vi "MasterAquisitionFile_IOS_Optogenetics_Test2.vi"() -> ()   [LabVIEW 2018]
uses:
  <vilib>/vision/driver/IMAQdx.llb/IMAQdx Camera Control Mode.ctl
  <vilib>/vision/driver/IMAQdx.llb/IMAQdx Acquisition Mode.ctl
  <vilib>/userdefined/High Color/IMAQdx.ctl
  <vilib>/vision/driver/IMAQdx.llb/IMAQdx Buffer Number Mode.ctl
  <vilib>/DAQmx/write.llb/DAQmx Write (Digital 1D Wfm NChan NSamp).vi
  <vilib>/DAQmx/read.llb/DAQmx Read (Analog 1D Wfm NChan NSamp).vi
  <vilib>/Waveform/DWDTOps.llb/DWDT Digital to Boolean Array.vi
  <vilib>/DAQmx/create/channels.llb/DAQmx Create Channel (CO-Pulse Generation-Frequency).vi
  <vilib>/DAQmx/configure/timing.llb/DAQmx Timing (Implicit).vi
  <vilib>/DAQmx/create/channels.llb/DAQmx Create Channel (AI-Voltage-Basic).vi
  <vilib>/DAQmx/configure/timing.llb/DAQmx Timing (Sample Clock).vi
  <vilib>/DAQmx/configure/trigger.llb/DAQmx Start Trigger (Digital Edge).vi
  <vilib>/DAQmx/create/channels.llb/DAQmx Create Channel (DO-Digital Output).vi
  <vilib>/Waveform/DWDTOps.llb/DWDT Uncompress Digital.vi
  <vilib>/DAQmx/miscellaneous.llb/DAQmx Fill In Error Info.vi
  <vilib>/vision/driver/NI_Vision_Acquisition_Software.lvlib
  <resource>/objmgr/imaqdx.rc
  <resource>/objmgr/daqmx.rc
panel:
  out "Samples Written to Channel":dbl
  out "LED":bool
  out "Auditory":bool
  out "RPad":bool
  out "LPad":bool
  out "Finished":bool
  in  "Generate Stimuli":bool=TRUE
  in  "Sol Stim Parameters":cluster{"Fs":dbl, "Samples":dbl}
  in  "LED Stim Parameters":cluster{"Fs":dbl, "Samples":dbl}
  in  "Sol Duty Cycle (%)":dbl=10.0
  in  "Sol Freq":dbl=1.0
  in  "Sol Dur (s)":dbl=1.0
  in  "LED Duty Cycle (%)":dbl=10.0
  in  "LED Freq":dbl=10.0
  in  "LED Dur (s)":dbl=2.0
  out "Stimulus Order":digitalwaveform[](graph)=[{"t0"=timestamp(0 s since 1904-01-01), "dt"=5e-05, "Y"={"transitions"=[], "data"=array18000000x1[18000000 elements]}}, {"t0"=timestamp(0 s since 1904-01-01), "dt"=5e-05, "Y"={"transitions"=[], "data"=array18000000x1[18000000 elements]}}, {"t0"=timestamp(0 s since 1904-01-01), "dt"=5e-05, "Y"={"transitions"=[], "data"=array18000000x1[18000000 elements]}}, {"t0"=timestamp(0 s since 1904-01-01), "dt"=5e-05, "Y"={"transitions"=[], "data"=array18000000x1[18000000 elements]}}]
  out "Solenoid Stim":digitalwaveform(graph)={"t0"=timestamp(0 s since 1904-01-01), "dt"=5e-05, "Y"={"transitions"=[], "data"=array20000x1[20000 elements]}}
  in  "Trial Offset (s)":dbl=15.0
  in  "Interstim (s)":dbl=30.0
  in  "Right Pad":dbl=1.0
  in  "Left Pad":dbl=1.0
  in  "Auditory":dbl=1.0
  in  "LED":dbl
  out "Dev2 Samples":i32=526603
  out "Dev2 Analog":bool=TRUE
  in  "Dev2 Analog Channels":string[](array[string])=["LD_BackScatter", "LD_Flow", "Opto_LED", "RPadSol", "AudSol", "Hippocampus", "EMG", "Cortical_RH"]
  out "?":T1(plugin-control)
  out "?":T1(plugin-control)
  out "?":T1(plugin-control)
  out "?":T1(plugin-control)
  in  "stop":bool
  out "CBV Cam":bool=TRUE
  out "Pupil Cam":bool=TRUE
  out "Whisk Cam":bool=TRUE
  out "Web Cam":bool=TRUE
  out "Dev1 Analog":bool=TRUE
  out "Web Cam Fs":dbl(knob)=29.14753443801158 scale=0.0..200.0
  out "CBV Cam":dbl(knob)=30.019685039370078 scale=0.0..200.0
  out "Whisk Cam Fs":dbl(knob)=150.04985044865404 scale=0.0..200.0
  out "Last Whisk\nBuffer 2":u32=789
  out "Pupil Cam Fs":dbl(knob)=29.985007496251875 scale=0.0..200.0
  out "Dropped 2":u32(slide) caption="Pupil Cam" scale=0.0..99.0
  in  "Exposure Time (microsec)":string="10000"
  out "Dev1 Samples":i32=526592
  in  "Dev1 Analog Channels":string[](array[string])=["Cortical_LH", "Force_Sensor", "LPadSol", "RPadSol", "AudSol", "Hippocampus", "EMG", "Cortical_RH"]
  in  "Analog Acquisition":cluster{"Analog Fs":u16}={"Analog Fs"=20000} {"Analog Fs" format="%0.0f"}
  in  "Sampling Rates":T2={"CBV Cam Fs"=30, "Whisk Cam Fs"=150, "Web Cam Fs"=15, "Pupil Cam Fs"=30}
  out "Notes Size":i32=8
  out "Notes Reversed":string[](array[string])=["Experimenter", "Animal ID", "Hemisphere", "Solenoid PSI", "Isoflurane time", "Session ID", "Amplifier Gain", "LED power (mW)"]
  out "Notes Array":string[](array[string])=["LED power (mW)", "Amplifier Gain", "Session ID", "Isoflurane time", "Solenoid PSI", "Hemisphere", "Animal ID", "Experimenter"]
  in  "Notes:":T3={"Experimenter"="Kevin", "Animal ID"="T182", "Hemisphere"="Both", "Solenoid PSI"="10", "Isoflurane time"="1030", "Session ID"="Imaging Session Two", "Amplifier Gain"="10000", "LED power (mW)"="0"}
  in  "Target Path":path=path "D:/T182/Imaging Session 2 - 20 Apr. 2021" caption="Final Save Location"
  out "Dropped":u32(slide) caption="Whisk Cam" scale=0.0..999.0
  out "Filename":string="210420_10_44_31"
  out "CBV Camera":bool
  out "Time Elapsed (Min)":cluster{dbl, dbl}(slide)={15.0, 0.43888776} scale=0.0..15.0 scale format="%#_2g"
  in  "Time (min)":dbl(knob)=15.0 min=0.5 max=20.0 step=0.5 scale=0.0..20.0 scale format="%#_2g"
  in  "Temp Path":path=path "D:/LabVIEW Streamed Data" caption="Temporary Path for Streamed Data"
  out "Last CBV\nBuffer":i32=789
  out "Last Whisk\nBuffer":u32=3948
  # "Stimuli"
  # "LPAD"
  # "RPAD"
  # "AUD"
  # "LED"
  # "Ratio"
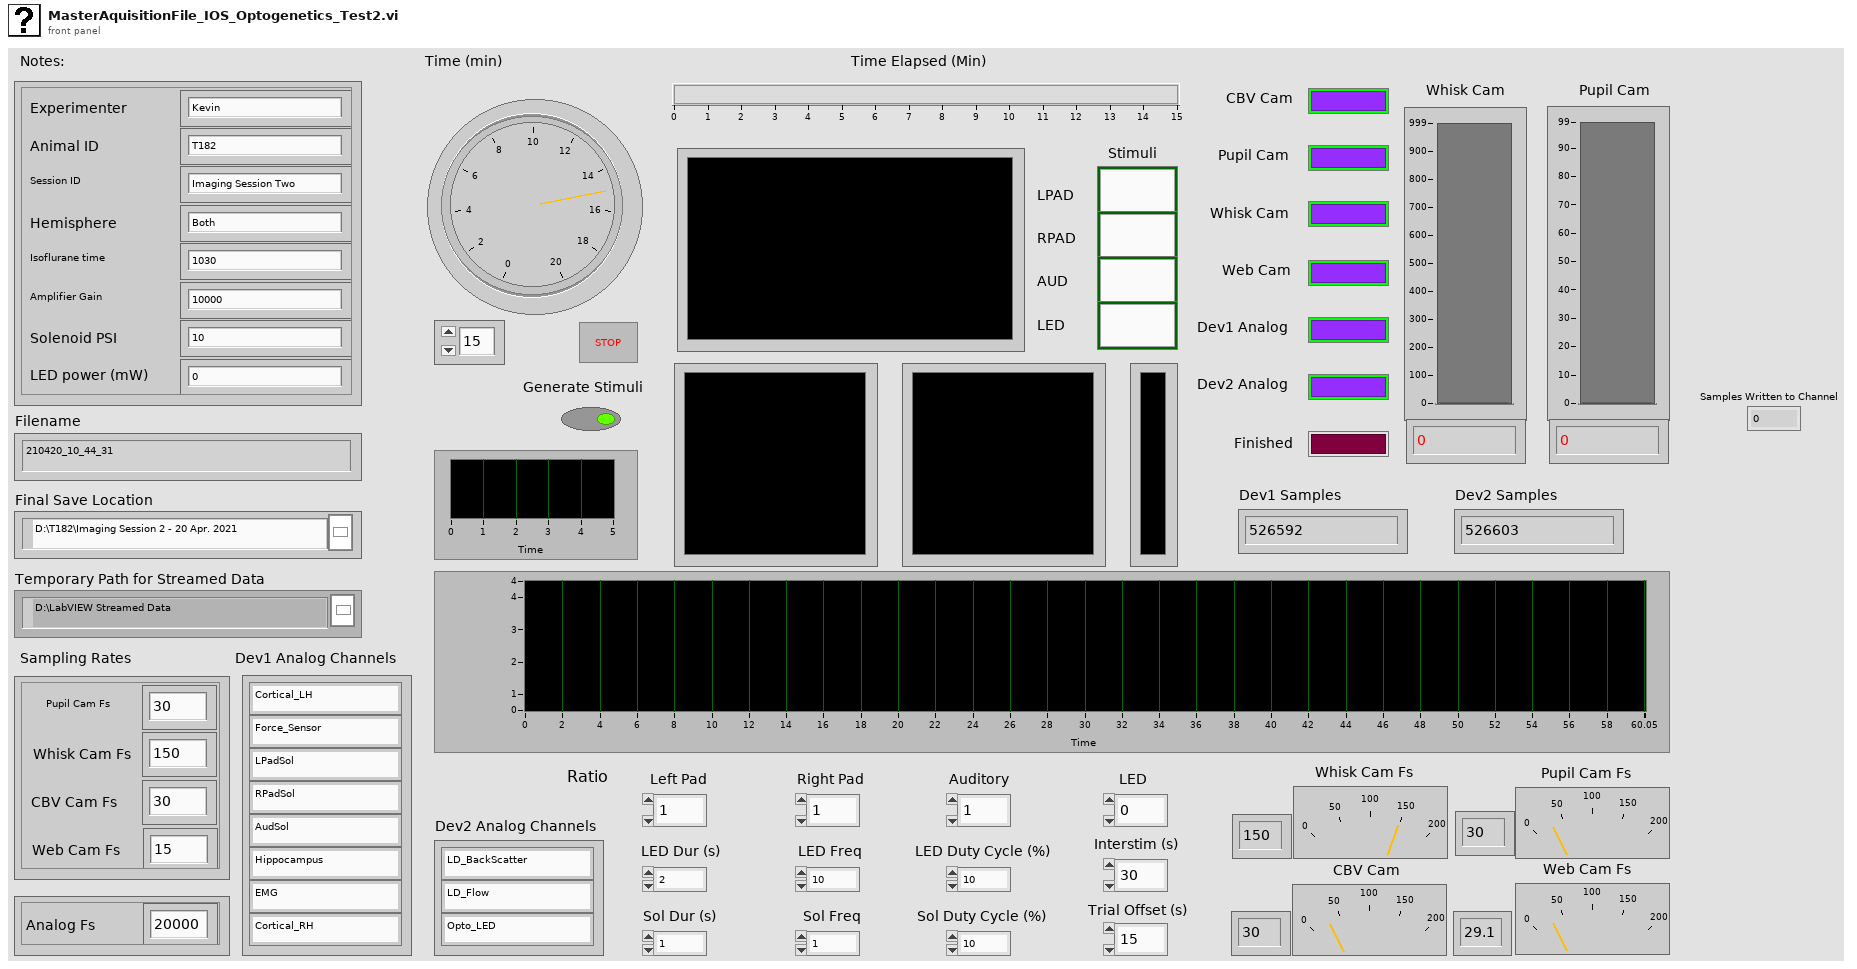
[diagram p1: front panel]
types:
  T1 = typedef "IMAQ Image.ctl" = refnum<image>
  T2 = cluster{"CBV Cam Fs":u16, "Whisk Cam Fs":u16, "Web Cam Fs":u16, "Pupil Cam Fs":u16}
  T3 = cluster{"Experimenter":string, "Animal ID":string, "Hemisphere":string, "Solenoid PSI":string, "Isoflurane time":string, "Session ID":string, "Amplifier Gain":string, "LED power (mW)":string}
  T4 = typedef "IMAQdx.ctl" = refnum<k21>
  T5 = enum16{"open", "open or create", "create or replace", "create", "open (read-only)"}
  T6 = enum16{"open", "replace", "create", "open or create", "replace or create", "replace or create with confirmation"}
  T7 = typedef "Image Type" = u32
  T8 = typedef "NI_Vision_Acquisition_Software.lvlib/IMAQdx Acquisition Mode.ctl" = enum32{"One Shot", "Continuous"}
  T9 = typedef "NI_Vision_Acquisition_Software.lvlib/IMAQdx Camera Control Mode.ctl" = enum32{"Controller", "Listener"}
  T10 = typedef "IMAQ AVI2 Refnum.ctl" = refnum<k20>
  T11 = enum16{"big-endian, network order", "native, host order", "little-endian"}
  T12 = typedef "NI_Vision_Acquisition_Software.lvlib/IMAQdx Buffer Number Mode.ctl" = enum32{"Next", "Last", "Buffer Number", "Every", "Last New"}
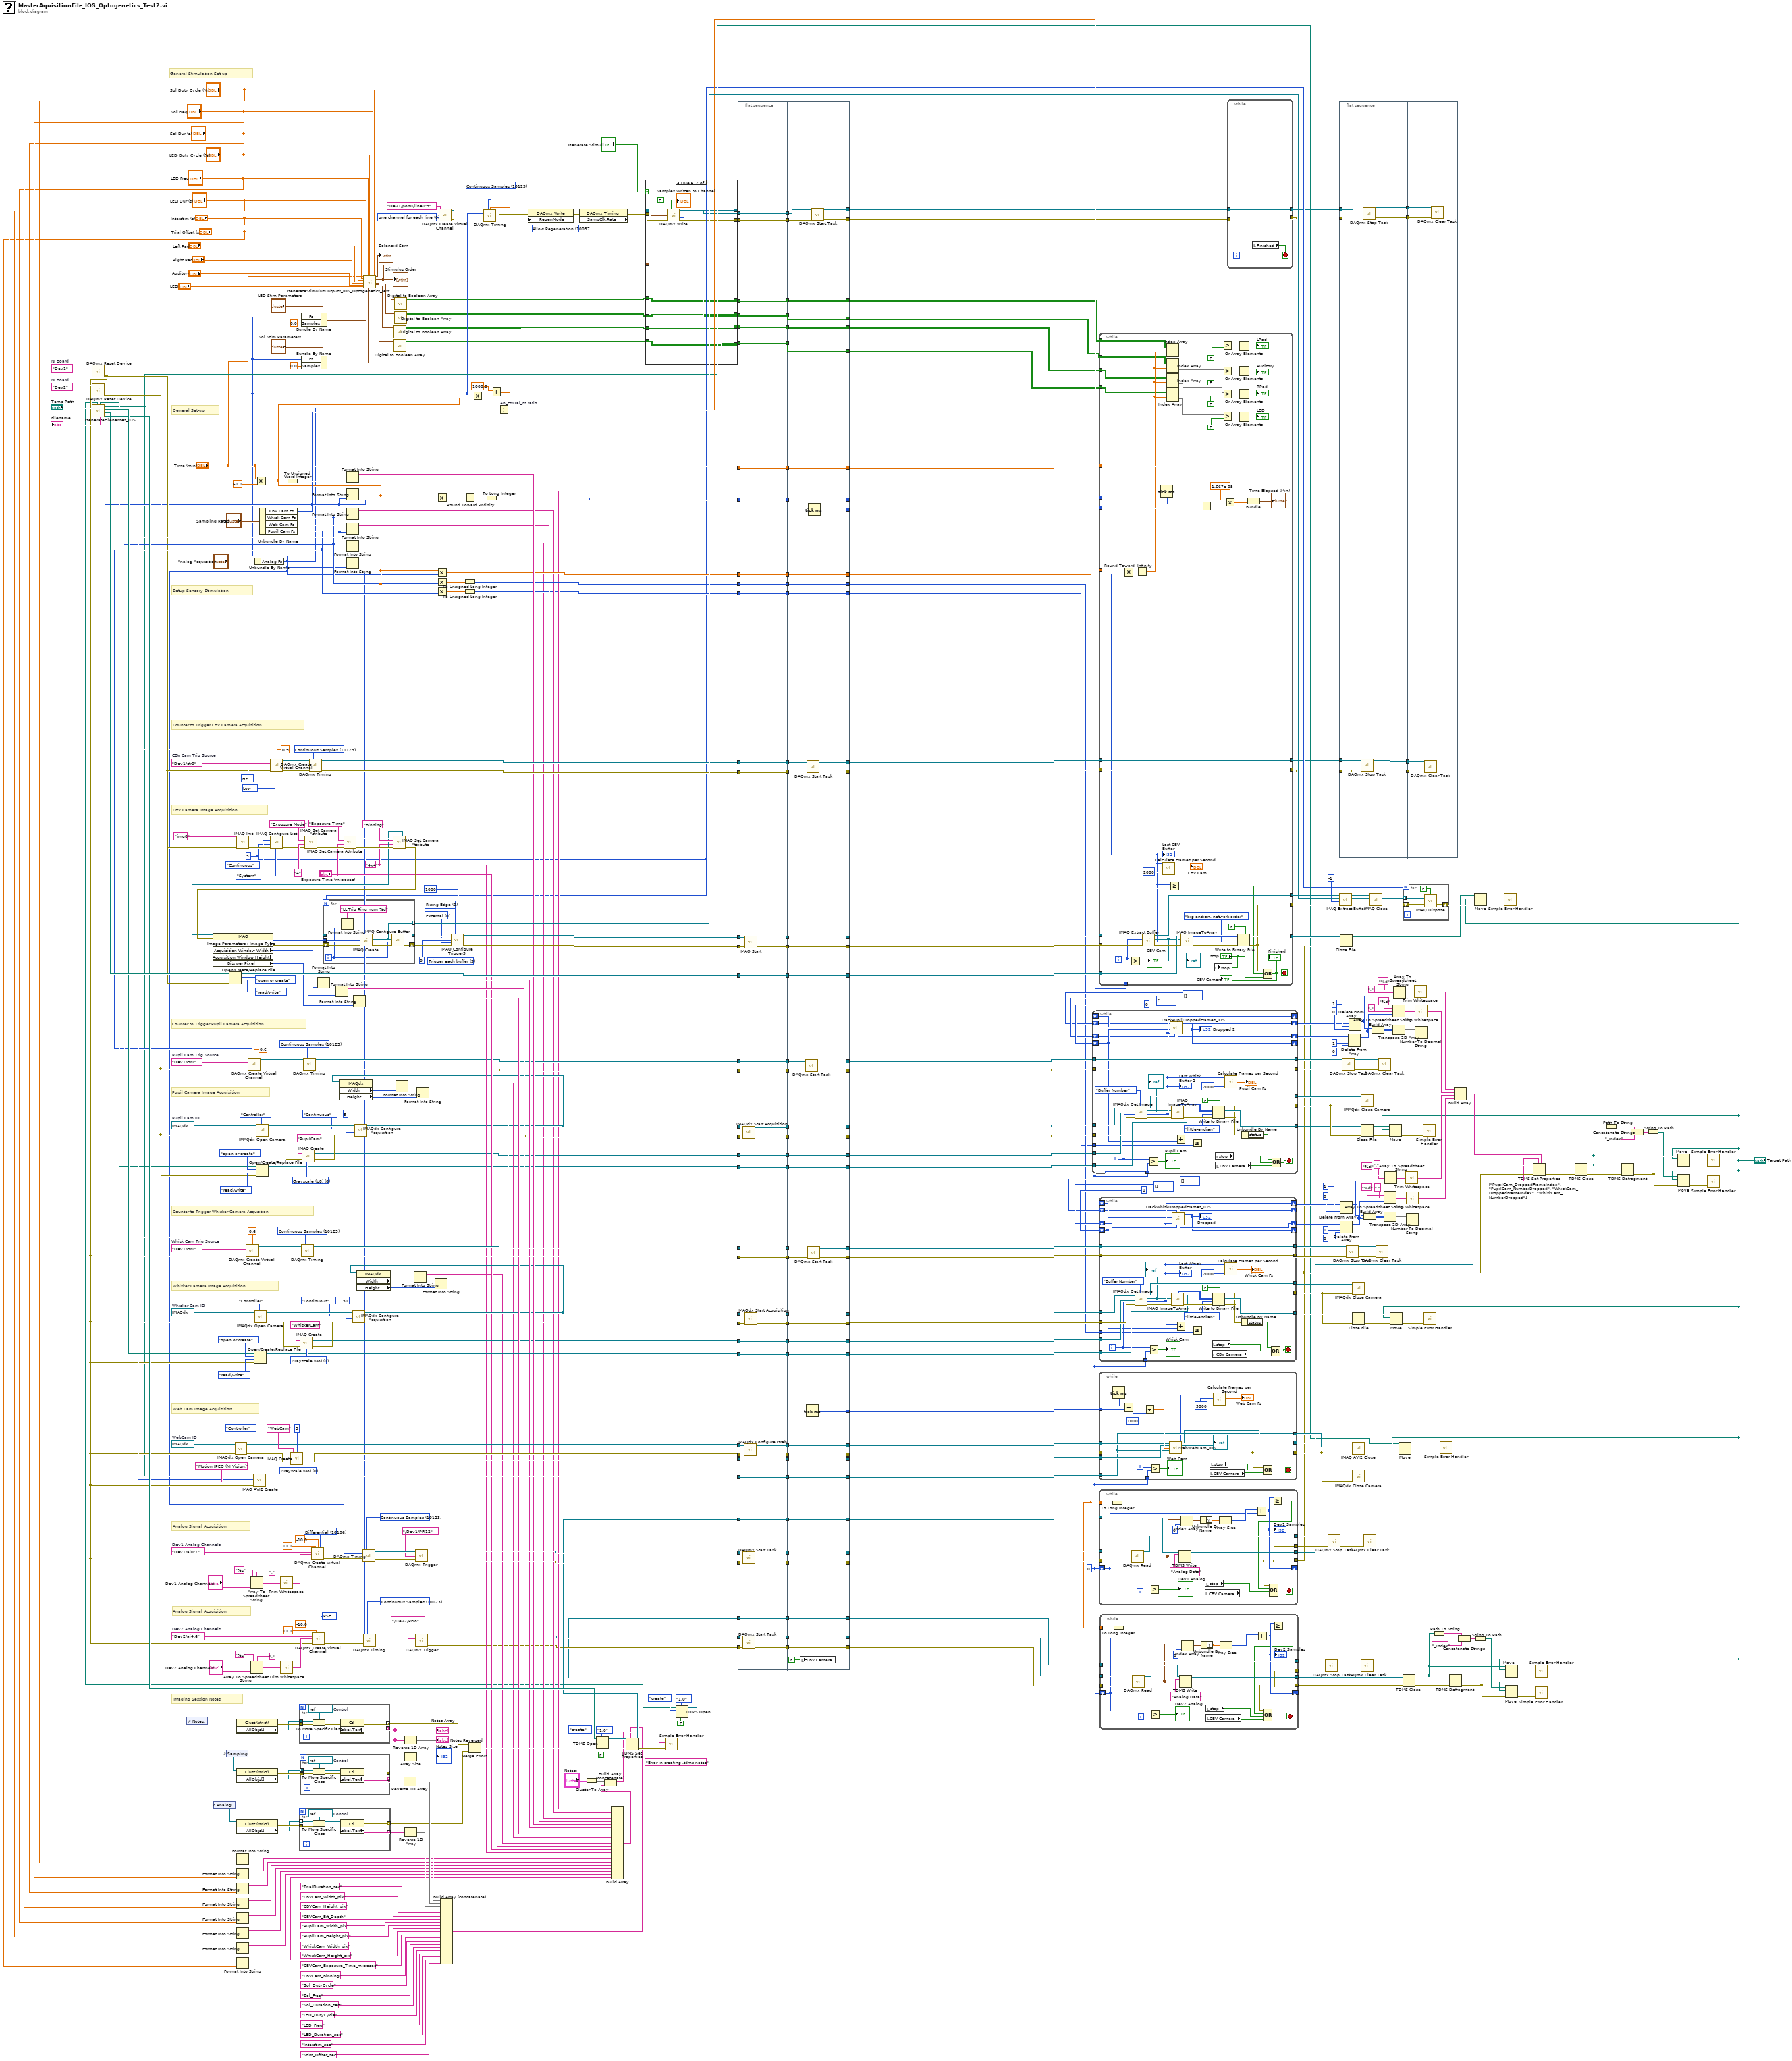
[diagram p0: block diagram]
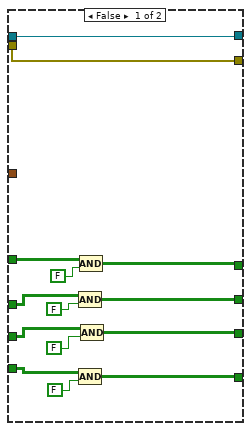
[diagram p2: hidden frame]
diagram:
  w35 = 10097 items=["Allow Regeneration"=10097, "Do Not Allow Regeneration"=10158] ("RegenMode")
  w36 = 10123 items=["Finite Samples"=10178, "Continuous Samples"=10123, "Hardware Timed Single Point"=12522] ("sample mode")
  w39 = 0 items=["one channel for each line", "one channel for all lines"] ("line grouping")
  w135 = tag "Dev2/ai4:6"  # Dev2 Analog Channels
  w315 = tag "Dev1/ai0:7"  # Dev1 Analog Channels
  w318 = T4 "cam0"  # WebCam ID
  w296 = T4 "cam1"  # Whisker Cam ID
  w488 = tag "Dev1/ctr1"  # Whisk Cam Trig Source
  w233 = T4 "cam2"  # Pupil Cam ID
  w238 = tag "Dev1/ctr0"  # Pupil Cam Trig Source
  w462 = tag "Dev1/ctr0"  # CBV Cam Trig Source
  w139 = 10123 items=["Finite Samples"=10178, "Continuous Samples"=10123, "Hardware Timed Single Point"=12522] ("sample mode")
  w142 = 10083 items=["default"=-1, "RSE"=10083, "NRSE"=10078, "Differential"=10106, "Pseudodifferential"=12529] ("input terminal configuration")
  w156 = tag "Dev2"  # NI Board
  w234 = 10123 items=["Finite Samples"=10178, "Continuous Samples"=10123, "Hardware Timed Single Point"=12522] ("sample mode")
  w241 = T7 0 items=["Grayscale (U8)", "Grayscale (I16)", "Grayscale (SGL)", "Complex (CSG)", "RGB (U32)", "HSL (U32)", "RGB (U64)", "Grayscale (U16)"] ("Image Type")
  w223 = "4x4" ("Attribute Value")
  w94 = 0
  w397 = 10123 items=["Finite Samples"=10178, "Continuous Samples"=10123, "Hardware Timed Single Point"=12522] ("sample mode")
  w400 = 10106 items=["default"=-1, "RSE"=10083, "NRSE"=10078, "Differential"=10106, "Pseudodifferential"=12529] ("input terminal configuration")
  w449 = T7 0 items=["Grayscale (U8)", "Grayscale (I16)", "Grayscale (SGL)", "Complex (CSG)", "RGB (U32)", "HSL (U32)", "RGB (U64)", "Grayscale (U16)"] ("Image Type")
  w469 = u32 0 items=["Rising Edge", "Falling Edge"] ("Trigger Polarity")
  w472 = u32 0 items=["External"=0, "RTSI"=1, "ISO In"=2, "Scaled Encoder"=5] ("Trigger Type")
  w463 = tag "Dev1"  # NI Board
  w464 = 10123 items=["Finite Samples"=10178, "Continuous Samples"=10123, "Hardware Timed Single Point"=12522] ("sample mode")
  w467 = 10373 items=["Hz"=10373] ("units")
  w468 = 10214 items=["High"=10192, "Low"=10214] ("idle state")
  w32 = u32 5 ("Number of Buffers")
  w470 = u32 3 items=["Disabled", "Trigger start of acquisition", "Trigger start of each buffer list", "Trigger each buffer", "Trigger each line (linescan)", "Trigger end of acquisition"] ("Action")
  w484 = 10123 items=["Finite Samples"=10178, "Continuous Samples"=10123, "Hardware Timed Single Point"=12522] ("sample mode")
  w491 = T7 0 items=["Grayscale (U8)", "Grayscale (I16)", "Grayscale (SGL)", "Complex (CSG)", "RGB (U32)", "HSL (U32)", "RGB (U64)", "Grayscale (U16)"] ("Image Type")
  # "General Stimulation Set-up"
  # "Analog Signal Acquisition"
  # "General Set-up"
  # "Pupil Camera Image Acquisition"
  # "Counter to Trigger Pupil Camera Acquisition"
  # "Whisker Camera Image Acquisition"
  # "Imaging Session Notes"
  # "Setup Sensory Stimulation"
  # "CBV Camera Image Acquisition"
  # "Counter to Trigger CBV Camera Acquisition"
  # "Counter to Trigger Whisker Camera Acqusition"
  # "Web Cam Image Acquisition"
  # "Analog Signal Acquisition"
  n1 = call <vilib>:"DAQmx Reset Device.vi"("device in"=w463) -> ("error out"=w128:errorcluster)  [unwired: 14 in]
  n2 = call <vilib>:"DAQmx Reset Device.vi"("device in"=w156) -> ("error out"=w155:errorcluster)  [unwired: 14 in]
  n3 = call "GenerateFilenames_IOS.vi"("path"="Temp Path") -> ("TDMS Path"=w340:path, "Dalsa Path"=w456:path, "Basler Path"=w452:path, "WebCam Path"=w79:path, "Analog file name"=→"Filename":string, "Basler2 Path"=w232:path, "TDMS Path 2"=w96:path)  [unwired: 3 in, 1 out]
  n4 = control-ref of="Notes:"() -> (w345:refnum<vi>)
  n5 = control-ref of="Analog Acquisition"() -> (w323:refnum<vi>)
  n6 = control-ref of="Sampling Rates"() -> (w324:refnum<vi>)
  n7 = Open/Create/Replace File(file path (use dialog)=w456, error in=w128, operation (0:open)=T6."open or create", access (0:read/write)=enum16{"read/write", "read-only", "write-only"}."read/write") -> (refnum out=w401:refnum<file>)  [unwired: 2 in, 2 out]
  n8 = call <vilib>:"IMAQdx Open Camera.vi"("Camera Control Mode"=IMAQdx_Camera_Control_Mode."Controller", "error in"=w128, "Session In"=w318) -> ("error out"=w445:errorcluster, "Session Out"=w443:T4)  [unwired: 7 in]
  n9 = property class="Clust (strict)"(reference=w345) -> (error out=w348:errorcluster, "AllObjs[]"=w258:refnum<vi>[])  [unwired: 1 in, 1 out]
  n10 = property class="Clust (strict)"(reference=w324) -> (error out=w343:errorcluster, "AllObjs[]"=w259:refnum<vi>[])  [unwired: 1 in, 1 out]
  n11 = property class="Clust (strict)"(reference=w323) -> (error out=w322:errorcluster, "AllObjs[]"=w257:refnum<vi>[])  [unwired: 1 in, 1 out]
  n12 = call <vilib>:"IMAQ Init.vi"("error in (no error)"=w128, "Interface Name"="img0") -> ("error out"=w482:errorcluster, "IMAQ Session Out"=w483:refnum<k11>)  [unwired: 8 out]
  n13 = Format Into String("Sol Duty Cycle (%)") -> (resulting string=w69:string)  [unwired: 3 in, 1 out]
  n14 = Format Into String("Sol Freq") -> (resulting string=w68:string)  [unwired: 3 in, 1 out]
  n15 = Format Into String("Sol Dur (s)") -> (resulting string=w67:string)  [unwired: 3 in, 1 out]
  n16 = Format Into String("LED Duty Cycle (%)") -> (resulting string=w66:string)  [unwired: 3 in, 1 out]
  n17 = Format Into String("LED Freq") -> (resulting string=w65:string)  [unwired: 3 in, 1 out]
  n18 = Format Into String("LED Dur (s)") -> (resulting string=w64:string)  [unwired: 3 in, 1 out]
  n19 = Format Into String("Interstim (s)") -> (resulting string=w63:string)  [unwired: 3 in, 1 out]
  n20 = Format Into String("Trial Offset (s)") -> (resulting string=w62:string)  [unwired: 3 in, 1 out]
  n21 = Array To Spreadsheet String(delimiter (Tab)=",", array="Dev1 Analog Channels", 3:"%s" ("format string")) -> (spreadsheet string=w312:string)
  n22 = Array To Spreadsheet String(delimiter (Tab)=",", array="Dev2 Analog Channels", 3:"%s" ("format string")) -> (spreadsheet string=w132:string)
  n23 = Open/Create/Replace File(file path (use dialog)=w452, error in=w128, operation (0:open)=T6."open or create", access (0:read/write)=enum16{"read/write", "read-only", "write-only"}."read/write") -> (refnum out=w417:refnum<file>)  [unwired: 2 in, 2 out]
  n24 = Unbundle By Name("Analog Acquisition") -> ("Analog Fs"=w52:u16)
  n25 = call <vilib>:"IMAQdx Open Camera.vi"("Camera Control Mode"=IMAQdx_Camera_Control_Mode."Controller", "error in"=w128, "Session In"=w296) -> ("error out"=w494:errorcluster, "Session Out"=w497:T4)  [unwired: 7 in]
  n26 = Multiply(x="Time (min)", y=60.0) -> (x*y=w80:dbl)
  n27 = Open/Create/Replace File(file path (use dialog)=w232, error in=w155, operation (0:open)=T6."open or create", access (0:read/write)=enum16{"read/write", "read-only", "write-only"}."read/write") -> (refnum out=w213:refnum<file>)  [unwired: 2 in, 2 out]
  n28 = call <vilib>:"IMAQdx Open Camera.vi"("Camera Control Mode"=IMAQdx_Camera_Control_Mode."Controller", "error in"=w155, "Session In"=w233) -> ("error out"=w244:errorcluster, "Session Out"=w247:T4)  [unwired: 7 in]
  n29 = Unbundle By Name("Sampling Rates") -> ("CBV Cam Fs"=w82:u16, "Whisk Cam Fs"=w195:u16, "Web Cam Fs"=w317:u16, "Pupil Cam Fs"=w189:u16)
  n30 = call-poly <vilib>:"DAQmx Create Virtual Channel.vi"("frequency"=w195, "duty cycle"=0.6, "counter"=w488, "error in"=w128) -> ("task out"=w486:refnum<k21>, "error out"=w485:errorcluster)  [unwired: 10 in]
  n31 = call-poly <vilib>:"DAQmx Create Virtual Channel.vi"("frequency"=w189, "duty cycle"=0.6, "counter"=w238, "error in"=w155) -> ("task out"=w236:refnum<k21>, "error out"=w235:errorcluster)  [unwired: 10 in]
  n32 = call "IMAQ AVI2 Create"("error in (no error)"=w128, "Codec"="Motion JPEG (NI Vision)", "Frames Per Second"=w317, "AVI Path"=w79) -> ("AVI Refnum"=w435:T10)  [unwired: 6 in, 1 out]
  n33 = call-poly <vilib>:"DAQmx Create Virtual Channel.vi"("frequency"=w82, "duty cycle"=0.9, "counter"=w462, "units"=w467, "error in"=w128, "idle state"=w468) -> ("task out"=w466:refnum<k21>, "error out"=w465:errorcluster)  [unwired: 8 in]
  n34 = call <vilib>:"IMAQ Configure List.vi"("Memory Location"=enum16{"System", "Onboard"}."System", "error in (no error)"=w482, "Number of buffers"=w32, "Continuous?"=enum16{"One-Shot", "Continuous"}."Continuous" ("Continuous ?"), "IMAQ Session In"=w483) -> ("error out"=w272:errorcluster, "IMAQ Session Out"=w268:refnum<k11>)  [unwired: 1 in, 4 out]
  n35 = call <vilib>:"Trim Whitespace.vi"("string"=w312) -> ("trimmed string"=w311:string)  [unwired: 1 in]
  n36 = call <vilib>:"Trim Whitespace.vi"("string"=w132) -> ("trimmed string"=w131:string)  [unwired: 1 in]
  n37 = To Unsigned Word Integer(number=w80) -> (unsigned 16bit integer=w307:u16)
  n38 = call "IMAQ Create"("Border Size"=3, "Image Name"="WebCam", "Image Type"=w449, "error in (no error)"=w445) -> ("New Image"=w442:T1, "error out"=w444:errorcluster)  [unwired: 1 in]
  n39 = for {
    tunnel: [w503] -> w347 mode=indexing
    tunnel: w348 -> [w502]
    tunnel: [w500] -> w331 mode=indexing
    tunnel: w258 -> [w499] mode=indexing
    w504 = refnum<vi> refnum  # Control
    n40 = To More Specific Class(target class=w504, reference=w499, error in=w502) -> (specific class reference=w505:refnum<vi>, error out=w501:errorcluster)
    n41 = property class="Ctl"(reference=w505, error in=w501) -> (error out=w500:errorcluster, "Label.Text"=w503:string)  [unwired: 1 out]
  }
  "Notes Array" <- w347
  n42 = for {
    tunnel: [w510] -> w320 mode=indexing
    tunnel: w322 -> [w509]
    tunnel: [w507] -> w321 mode=indexing
    tunnel: w257 -> [w506] mode=indexing
    w511 = refnum<vi> refnum  # Control
    n43 = To More Specific Class(target class=w511, reference=w506, error in=w509) -> (specific class reference=w512:refnum<vi>, error out=w508:errorcluster)
    n44 = property class="Ctl"(reference=w512, error in=w508) -> (error out=w507:errorcluster, "Label.Text"=w510:string)  [unwired: 1 out]
  }
  n45 = call "IMAQ Create"("Image Name"="WhiskerCam", "Image Type"=w491, "error in (no error)"=w494) -> ("New Image"=w294:T1, "error out"=w492:errorcluster)  [unwired: 2 in]
  n46 = for {
    tunnel: [w517] -> w344 mode=indexing
    tunnel: w343 -> [w516]
    tunnel: [w514] -> w330 mode=indexing
    tunnel: w259 -> [w513] mode=indexing
    w518 = refnum<vi> refnum  # Control
    n47 = To More Specific Class(target class=w518, reference=w513, error in=w516) -> (specific class reference=w519:refnum<vi>, error out=w515:errorcluster)
    n48 = property class="Ctl"(reference=w519, error in=w515) -> (error out=w514:errorcluster, "Label.Text"=w517:string)  [unwired: 1 out]
  }
  n49 = Bundle By Name(cluster="LED Stim Parameters", "Fs"=w52, "Samples"=0.0) -> (w87:cluster{"Fs":dbl, "Samples":dbl})
  n50 = Bundle By Name(cluster="Sol Stim Parameters", "Fs"=w52, "Samples"=0.0) -> (w88:cluster{"Fs":dbl, "Samples":dbl})
  n51 = call-poly <vilib>:"DAQmx Timing.vi"("task/channels in"=w486, "sample mode"=w484, "error in"=w485) -> ("task out"=w382:refnum<k21>, "error out"=w380:errorcluster)  [unwired: 11 in]
  n52 = call "IMAQ Create"("Image Name"="PupilCam", "Image Type"=w241, "error in (no error)"=w244) -> ("New Image"=w198:T1, "error out"=w242:errorcluster)  [unwired: 2 in]
  n53 = call-poly <vilib>:"DAQmx Timing.vi"("task/channels in"=w236, "sample mode"=w234, "error in"=w235) -> ("task out"=w211:refnum<k21>, "error out"=w209:errorcluster)  [unwired: 11 in]
  n54 = call <vilib>:"IMAQ Set Camera Attribute.vi"("error in (no error)"=w272, "Attribute Value"="4", "Camera Attribute"="Exposure Mode", "IMAQ Session In"=w268) -> ("error out"=w271:errorcluster, "IMAQ Session Out"=w267:refnum<k11>)  [unwired: 4 in]
  n55 = call-poly <vilib>:"DAQmx Timing.vi"("task/channels in"=w466, "sample mode"=w464, "error in"=w465) -> ("task out"=w386:refnum<k21>, "error out"=w384:errorcluster)  [unwired: 11 in]
  n56 = call-poly <vilib>:"DAQmx Create Virtual Channel.vi"("maximum value"=10.0, "minimum value"=-10.0, "input terminal configuration"=w400, "physical channels"=w315, "name to assign"=w311, "error in"=w128) -> ("task out"=w399:refnum<k21>, "error out"=w398:errorcluster)  [unwired: 8 in]
  n57 = call-poly <vilib>:"DAQmx Create Virtual Channel.vi"("maximum value"=10.0, "minimum value"=-10.0, "input terminal configuration"=w142, "physical channels"=w135, "name to assign"=w131, "error in"=w128) -> ("task out"=w141:refnum<k21>, "error out"=w140:errorcluster)  [unwired: 8 in]
  n58 = call <vilib>:"IMAQ Set Camera Attribute.vi"("error in (no error)"=w271, "Attribute Value"="Exposure Time (microsec)", "Camera Attribute"="Exposure Time", "IMAQ Session In"=w267) -> ("error out"=w270:errorcluster, "IMAQ Session Out"=w266:refnum<k11>)  [unwired: 4 in]
  n59 = Format Into String(w307) -> (resulting string=w309:string)  [unwired: 3 in, 1 out]
  n60 = Format Into String(w82) -> (resulting string=w193:string)  [unwired: 3 in, 1 out]
  n61 = Format Into String(w195) -> (resulting string=w192:string)  [unwired: 3 in, 1 out]
  n62 = Format Into String(w317) -> (resulting string=w191:string)  [unwired: 3 in, 1 out]
  n63 = Format Into String(w189) -> (resulting string=w144:string)  [unwired: 3 in, 1 out]
  n64 = Format Into String(w52) -> (resulting string=w143:string)  [unwired: 3 in, 1 out]
  n65 = call <vilib>:"IMAQdx Configure Acquisition.vi"("error in"=w492, "Number of Buffers"=u32 50, "Continuous?"=IMAQdx_Acquisition_Mode."Continuous", "Session In"=w497) -> ("error out"=w157:errorcluster, "Session Out"=w295:T4)  [unwired: 6 in]
  n66 = call <vilib>:"IMAQdx Configure Acquisition.vi"("error in"=w242, "Number of Buffers"=u32 5, "Continuous?"=IMAQdx_Acquisition_Mode."Continuous", "Session In"=w247) -> ("error out"=w215:errorcluster, "Session Out"=w199:T4)  [unwired: 6 in]
  n67 = property class="IMAQdx"(reference=w199) -> ("Width"=w231:u32, "Height"=w230:u32)  [unwired: 1 in, 2 out]
  n68 = property class="IMAQdx"(reference=w295) -> ("Width"=w306:u32, "Height"=w305:u32)  [unwired: 1 in, 2 out]
  n69 = call-poly <vilib>:"DAQmx Timing.vi"("task/channels in"=w399, "sample mode"=w397, "rate"=w52, "error in"=w398) -> ("task out"=w255:refnum<k21>, "error out"=w396:errorcluster)  [unwired: 10 in]
  n70 = call-poly <vilib>:"DAQmx Timing.vi"("task/channels in"=w141, "sample mode"=w139, "rate"=w52, "error in"=w140) -> ("task out"=w129:refnum<k21>, "error out"=w138:errorcluster)  [unwired: 10 in]
  n71 = call "GenerateStimulusOutputs_IOS_Optogenetics_test.vi"("Trial duration (min)"="Time (min)", "Rest duration(s)"="Interstim (s)", "trial offset (s)"="Trial Offset (s)", "Left Pad"="Left Pad", "Right Pad"="Right Pad", "Auditory"="Auditory", "LED"="LED", "LED Stim Duration (s)"="LED Dur (s)", "LED Stim Parameters"=w87, "LED Frequency"="LED Freq", "Sol Stim Parameters"=w88, "LED duty cycle (%)"="LED Duty Cycle (%)", "Sol Stim Duration (s)"="Sol Dur (s)", "Sol Frequency"="Sol Freq", "Sol Duty Cycle (%)"="Sol Duty Cycle (%)") -> ("Solenoid Stim Waveforms"=→"Solenoid Stim":digitalwaveform, "Stimulus Digital Outputs"=w12:digitalwaveform[], "Left Pad Out"=w43:digitalwaveform, "Auditory Out"=w42:digitalwaveform, "Right Pad Out"=w41:digitalwaveform, "LED Out"=w40:digitalwaveform)  [unwired: 3 in, 4 out]
  "Stimulus Order" <- w12
  n72 = call <vilib>:"IMAQ Set Camera Attribute.vi"("error in (no error)"=w270, "Attribute Value"=w223, "Camera Attribute"="Binning", "IMAQ Session In"=w266) -> ("error out"=w269:errorcluster, "IMAQ Session Out"=w265:refnum<k11>)  [unwired: 4 in]
  n73 = property class="IMAQ"(reference=w265, error in=w269) -> (reference out=w279:refnum<k11>, error out=w278:errorcluster, "Image Parameters : Image Type"=w478:u32, "Acquisition Window Width"=w304:u32, "Acquisition Window Height"=w303:u32, "Bits per Pixel"=w302:u32)
  n74 = Format Into String(w304) -> (resulting string=w301:string)  [unwired: 3 in, 1 out]
  n75 = for {
    N: w32 -> [_]
    tunnel: [w529] -> w474
    tunnel: w478 -> [w527]
    shift-right: [w528] -> w473
    shift-left: w278 -> [w526]
    tunnel: [w521] -> w475 mode=indexing
    tunnel: w279 -> [w520]
    i -> [w522]
    n76 = Format Into String(format string="LL Trig Ring num %d", w522) -> (resulting string=w524:string)  [unwired: 2 in, 1 out]
    n77 = call "IMAQ Create"("Image Name"=w524, "Image Type"=w527, "error in (no error)"=w526) -> ("New Image"=w521:T1, "error out"=w525:errorcluster)  [unwired: 1 in, 1 out]
    n78 = call <vilib>:"IMAQ Configure Buffer.vi"("error in (no error)"=w525, "Buffer Number"=w522, "Image In"=w521, "IMAQ Session In"=w520) -> ("error out"=w528:errorcluster, "IMAQ Session Out"=w529:refnum<k11>)  [unwired: 2 in, 4 out]
  }
  n79 = Format Into String(w303) -> (resulting string=w252:string)  [unwired: 3 in, 1 out]
  n80 = Format Into String(w302) -> (resulting string=w300:string)  [unwired: 3 in, 1 out]
  n81 = call-poly <vilib>:"Digital to Boolean Array.vi"("digital waveform"=w41) -> ("boolean array"=w18:bool[][])  [unwired: 9 in, 1 out]
  n82 = call-poly <vilib>:"Digital to Boolean Array.vi"("digital waveform"=w40) -> ("boolean array"=w17:bool[][])  [unwired: 9 in, 1 out]
  n83 = call-poly <vilib>:"Digital to Boolean Array.vi"("digital waveform"=w43) -> ("boolean array"=w20:bool[][])  [unwired: 9 in, 1 out]
  n84 = call-poly <vilib>:"Digital to Boolean Array.vi"("digital waveform"=w42) -> ("boolean array"=w19:bool[][])  [unwired: 9 in, 1 out]
  n85 = Format Into String(w231) -> (resulting string=w218:string)  [unwired: 3 in, 1 out]
  n86 = Reverse 1D Array(array=w344) -> (reversed array=w334:string[])
  n87 = Reverse 1D Array(array=w347) -> (reversed array=w256:string[])
  "Notes Reversed" <- w256
  n88 = Array Size(array=w347) -> (size(s)=→"Notes Size":i32)
  n89 = Reverse 1D Array(array=w320) -> (reversed array=w319:string[])
  n90 = Format Into String(w306) -> (resulting string=w220:string)  [unwired: 3 in, 1 out]
  n91 = call-poly <vilib>:"DAQmx Trigger.vi"("task/channels in"=w255, "source"=tag "/Dev1/PFI12", "error in"=w396) -> ("task out"=w395:refnum<k21>, "error out"=w394:errorcluster)  [unwired: 11 in]
  n92 = call-poly <vilib>:"DAQmx Trigger.vi"("task/channels in"=w129, "source"=tag "/Dev2/PFI8", "error in"=w138) -> ("task out"=w127:refnum<k21>, "error out"=w126:errorcluster)  [unwired: 11 in]
  n93 = Format Into String(w230) -> (resulting string=w219:string)  [unwired: 3 in, 1 out]
  n94 = Format Into String(w305) -> (resulting string=w221:string)  [unwired: 3 in, 1 out]
  n95 = Multiply(x=w80, y=w82) -> (x*y=w454:dbl)
  n96 = Multiply(x=w80, y=w52) -> (x*y=w283:dbl)
  n97 = Multiply(x=w195, y=w80) -> (x*y=w253:dbl)
  n98 = Multiply(x=w189, y=w80) -> (x*y=w194:dbl)
  n99 = call-poly <vilib>:"DAQmx Create Virtual Channel.vi"("lines"=tag "Dev1/port0/line0:3", "line grouping"=w39) -> ("task out"=w38:refnum<k21>, "error out"=w37:errorcluster)  [unwired: 12 in]
  n100 = Build Array (concatenate)(w256, w334, w319, "TrialDuration_sec", "CBVCam_Width_pix", "CBVCam_Height_pix", "CBVCam_Bit_Depth", "PupilCam_Width_pix", "PupilCam_Height_pix", "WhiskCam_Width_pix", "WhiskCam_Height_pix", "CBVCam_Exposure_Time_microsec" ("element"), "CBVCam_Binning" ("element"), "Sol_DutyCycle", "Sol_Freq", "Sol_Duration_sec", "LED_DutyCycle", "LED_Freq", "LED_Duration_sec", "Interstim_sec", "Stim_Offset_sec") -> (w249:string[])
  n101 = call <vilib>:"IMAQ Configure Trigger3.vi"("IMAQ Session In"=w474, "Polarity"=w469, "Frame timeout (ms)"=u32 1000 ("Frame Timeout (ms)"), "Type"=w472, "Line Number"=u32 0 ("Trigger Line Number"), "Action"=w470, "error in (no error)"=w473) -> ("IMAQ Session Out"=w416:refnum<k11>, "error out"=w415:errorcluster)  [unwired: 2 in, 5 out]
  n102 = To Unsigned Long Integer(number=w253) -> (unsigned 32bit integer=w281:u32)
  n103 = To Unsigned Long Integer(number=w194) -> (unsigned 32bit integer=w190:u32)
  n104 = Round Toward -Infinity(1:w454) -> (0:w453:dbl)
  n105 = Merge Errors(w331, w330, w321) -> (w329:errorcluster)
  n106 = Multiply(x=w52, y=w80) -> (x*y=w11:dbl)
  n107 = To Long Integer(number=w453) -> (32bit integer=w158:i32)
  n108 = Add(x=1000.0, y=w11) -> (x+y=w9:dbl)
  n109 = call-poly <vilib>:"DAQmx Timing.vi"("task/channels in"=w38, "sample mode"=w36, "samples per channel"=w9, "rate"=w52, "error in"=w37) -> ("task out"=w31:refnum<k21>, "error out"=w30:errorcluster)  [unwired: 9 in]
  n110 = Divide "An_Fs/Dal_Fs ratio"(x=w52, y=w82) -> (x/y=w81:dbl)
  n111 = property class="DAQmx Write"(reference=w31, error in=w30, "RegenMode"=w35) -> (reference out=w33:refnum<k21>, error out=w34:errorcluster)
  n112 = property class="DAQmx Timing" props=["SampClk.Rate"](reference=w33, error in=w34) -> (reference out=w28:refnum<k21>, error out=w27:errorcluster)  [unwired: 1 out]
  n113 = Cluster To Array(cluster="Notes:") -> (array=w341:string[])
  n114 = TDMS Open(6:FALSE ("disable buffering? (T)"), 7:enum16{"1.0", "2.0"}."1.0" ("file format version (2.0)"), 8:w329, 10:T5."create" ("operation (0:open)"), 11:w340) -> (0:w335:errorcluster, 3:w336:refnum<k34>)  [unwired: 2 in]
  n115 = Build Array(w193, w192, w191, w144, w143, w309, w301, w252, w300, w218, w219, w220, w221, "Exposure Time (microsec)", w223, w69, w68, w67, w66, w65, w64, w63, w62) -> (w316:string[])
  n116 = Build Array (concatenate)(w341, w316) -> (w333:string[])
  n117 = TDMS Set Properties(5:w333, 7:w249, 8:w335, 11:w336) -> (0:w328:errorcluster, 3:w332:refnum<k34>)  [unwired: 2 in, 2 out]
  n118 = case shown="True" "Generate Stimuli" {
    tunnel: w28 -> [w543 w554]
    tunnel: w27 -> [w542 w553]
    tunnel: [w543 w552] -> w25
    tunnel: [w542 w551] -> w23
    tunnel: w20 -> [w534 w550]
    tunnel: w19 -> [w535 w549]
    tunnel: w18 -> [w536 w548]
    tunnel: w17 -> [w537 w547]
    tunnel: [w541 w550] -> w16
    tunnel: [w540 w549] -> w15
    tunnel: [w539 w548] -> w14
    tunnel: [w538 w547] -> w13
    tunnel: w12 -> [_ w546]
    frame False {
      n119 = Compound Arithmetic op=AND(w535, FALSE) -> (w540:bool[][])
      n120 = Compound Arithmetic op=AND(w537, FALSE) -> (w538:bool[][])
      n121 = Compound Arithmetic op=AND(w534, FALSE) -> (w541:bool[][])
      n122 = Compound Arithmetic op=AND(w536, FALSE) -> (w539:bool[][])
    }
    frame True {
      n123 = call-poly <vilib>:"DAQmx Write.vi"("task/channels in"=w554, "auto start"=FALSE, "data"=w546, "error in"=w553) -> ("task out"=w552:refnum<k21>, "number of samples written per channel"=→"Samples Written to Channel":u32, "error out"=w551:errorcluster)  [unwired: 9 in]
    }
  }
  n124 = call <vilib>:"Simple Error Handler.vi"("error source (\" \")"="Error in creating .tdms notes" ("error source (\" \")"), "error in (no error)"=w328) -> ()  [unwired: 3 in, 5 out]
  n125 = TDMS Open(6:FALSE ("disable buffering? (T)"), 7:enum16{"1.0", "2.0"}."1.0" ("file format version (2.0)"), 10:T5."create" ("operation (0:open)"), 11:w96) -> (3:w99:refnum<k34>)  [unwired: 3 in, 1 out]
  n126 = flat-sequence {
    tunnel: w444 -> [w604]
    tunnel: w443 -> [w603]
    tunnel: w442 -> [w602]
    tunnel: [w602] -> w441
    tunnel: [w601] -> w439
    tunnel: [w600] -> w437
    tunnel: w435 -> [w599]
    tunnel: [w599] -> w434
    tunnel: w295 -> [w598]
    tunnel: w157 -> [w597]
    tunnel: [w596] -> w424
    tunnel: [w595] -> w422
    tunnel: [w594] -> w420
    tunnel: w294 -> [w594]
    tunnel: [w593] -> w418
    tunnel: w417 -> [w593]
    tunnel: w416 -> [w592]
    tunnel: w415 -> [w591]
    tunnel: [w590] -> w413
    tunnel: [w589] -> w411
    tunnel: w158 -> [w588]
    tunnel: [w588] -> w407
    tunnel: "Time (min)" -> [w587]
    tunnel: [w587] -> w404
    tunnel: [w586] -> w402
    tunnel: w401 -> [w586]
    tunnel: w395 -> [w585]
    tunnel: w394 -> [w584]
    tunnel: [w583] -> w393
    tunnel: [w582] -> w392
    tunnel: [w581] -> w388
    tunnel: w332 -> [w581]
    tunnel: w386 -> [w580]
    tunnel: [w580] -> w385
    tunnel: w384 -> [w579]
    tunnel: [w579] -> w383
    tunnel: w382 -> [w578]
    tunnel: [w578] -> w381
    tunnel: w380 -> [w577]
    tunnel: [w577] -> w379
    tunnel: w283 -> [w576]
    tunnel: [w576] -> w282
    tunnel: w281 -> [w575]
    tunnel: [w575] -> w280
    tunnel: [w568] -> w217
    tunnel: w199 -> [w569]
    tunnel: [w566] -> w216
    tunnel: w215 -> [w567]
    tunnel: [w574] -> w214
    tunnel: w213 -> [w574]
    tunnel: [w573] -> w212
    tunnel: w211 -> [w573]
    tunnel: [w572] -> w210
    tunnel: w209 -> [w572]
    tunnel: w198 -> [w571]
    tunnel: [w571] -> w197
    tunnel: w190 -> [w570]
    tunnel: [w570] -> w188
    tunnel: w127 -> [w565]
    tunnel: w126 -> [w564]
    tunnel: [w563] -> w125
    tunnel: [w562] -> w124
    tunnel: w99 -> [w561]
    tunnel: [w561] -> w98
    tunnel: [w560] -> w51
    tunnel: w16 -> [w560]
    tunnel: [w559] -> w50
    tunnel: w15 -> [w559]
    tunnel: [w558] -> w49
    tunnel: w14 -> [w558]
    tunnel: [w557] -> w48
    tunnel: w13 -> [w557]
    tunnel: [w556] -> w26
    tunnel: w25 -> [w556]
    tunnel: [w555] -> w24
    tunnel: w23 -> [w555]
    tunnel: [w653] -> w446
    tunnel: w441 -> [w652]
    tunnel: [w652] -> w440
    tunnel: w439 -> [w651]
    tunnel: [w651] -> w438
    tunnel: w437 -> [w650]
    tunnel: [w650] -> w436
    tunnel: w434 -> [w649]
    tunnel: [w649] -> w433
    tunnel: [w631] -> w430
    tunnel: [w630] -> w428
    tunnel: [w648] -> w425
    tunnel: w424 -> [w648]
    tunnel: [w647] -> w423
    tunnel: w422 -> [w647]
    tunnel: [w646] -> w421
    tunnel: w420 -> [w646]
    tunnel: [w645] -> w419
    tunnel: w418 -> [w645]
    tunnel: [w644] -> w414
    tunnel: w413 -> [w644]
    tunnel: [w643] -> w412
    tunnel: w411 -> [w643]
    tunnel: [w635] -> w410
    tunnel: [w634] -> w409
    tunnel: [w642] -> w408
    tunnel: w407 -> [w641]
    tunnel: [w641] -> w406
    tunnel: [w640] -> w405
    tunnel: w404 -> [w640]
    tunnel: [w639] -> w403
    tunnel: w402 -> [w639]
    tunnel: [w638] -> w390
    tunnel: w393 -> [w638]
    tunnel: [w637] -> w391
    tunnel: w392 -> [w637]
    tunnel: [w636] -> w122
    tunnel: w388 -> [w636]
    tunnel: w385 -> [w633]
    tunnel: w383 -> [w632]
    tunnel: w381 -> [w629]
    tunnel: w379 -> [w628]
    tunnel: w282 -> [w627]
    tunnel: [w627] -> w123
    tunnel: w280 -> [w626]
    tunnel: [w626] -> w187
    tunnel: w217 -> [w624]
    tunnel: w216 -> [w623]
    tunnel: w214 -> [w622]
    tunnel: w212 -> [w619]
    tunnel: w210 -> [w618]
    tunnel: [w616] -> w205
    tunnel: [w617] -> w204
    tunnel: [w624] -> w203
    tunnel: [w623] -> w202
    tunnel: [w622] -> w201
    tunnel: [w621] -> w196
    tunnel: w197 -> [w621]
    tunnel: [w620] -> w186
    tunnel: w188 -> [w620]
    tunnel: [w615] -> w120
    tunnel: w125 -> [w615]
    tunnel: [w614] -> w121
    tunnel: w124 -> [w614]
    tunnel: [w613] -> w97
    tunnel: w98 -> [w613]
    tunnel: w51 -> [w609]
    tunnel: w50 -> [w612]
    tunnel: w49 -> [w611]
    tunnel: w48 -> [w610]
    tunnel: [w609] -> w47
    tunnel: [w612] -> w46
    tunnel: [w611] -> w45
    tunnel: [w610] -> w44
    tunnel: w26 -> [w608]
    tunnel: w24 -> [w607]
    tunnel: [w606] -> w22
    tunnel: [w605] -> w21
    frame #0 {
      n127 = call <vilib>:"IMAQdx Start Acquisition.vi"("error in"=w567, "Session In"=w569) -> ("error out"=w566:errorcluster, "Session Out"=w568:T4)  [unwired: 8 in]
      n128 = call <vilib>:"DAQmx Start Task.vi"("task/channels in"=w585, "error in"=w584) -> ("task out"=w583:refnum<k21>, "error out"=w582:errorcluster)  [unwired: 12 in]
      n129 = call <vilib>:"DAQmx Start Task.vi"("task/channels in"=w565, "error in"=w564) -> ("task out"=w562:refnum<k21>, "error out"=w563:errorcluster)  [unwired: 12 in]
      n130 = call <vilib>:"IMAQdx Configure Grab.vi"("error in"=w604, "Session In"=w603) -> ("error out"=w600:errorcluster, "Session Out"=w601:T4)  [unwired: 8 in]
      n131 = call <vilib>:"IMAQ Start.vi"("error in (no error)"=w591, "IMAQ Session In"=w592) -> ("error out"=w589:errorcluster, "IMAQ Session Out"=w590:refnum<k11>)  [unwired: 8 out]
      n132 = call <vilib>:"IMAQdx Start Acquisition.vi"("error in"=w597, "Session In"=w598) -> ("error out"=w595:errorcluster, "Session Out"=w596:T4)  [unwired: 8 in]
    }
    frame #1 {
      n133 = local write "CBV Camera"(FALSE ("Finished Acquiring")) -> ()
      n134 = call <vilib>:"DAQmx Start Task.vi"("task/channels in"=w619, "error in"=w618) -> ("task out"=w616:refnum<k21>, "error out"=w617:errorcluster)  [unwired: 12 in]
      n135 = Tick Count (ms)() -> (millisecond timer value=w653:u32)
      n136 = call <vilib>:"DAQmx Start Task.vi"("task/channels in"=w633, "error in"=w632) -> ("task out"=w635:refnum<k21>, "error out"=w634:errorcluster)  [unwired: 12 in]
      n137 = call <vilib>:"DAQmx Start Task.vi"("task/channels in"=w629, "error in"=w628) -> ("task out"=w631:refnum<k21>, "error out"=w630:errorcluster)  [unwired: 12 in]
      n138 = Tick Count (ms)() -> (millisecond timer value=w642:u32)
      n139 = call <vilib>:"DAQmx Start Task.vi"("task/channels in"=w608, "error in"=w607) -> ("task out"=w606:refnum<k21>, "error out"=w605:errorcluster)  [unwired: 12 in]
    }
  }
  n140 = while {
    tunnel: w205 -> [w679]
    tunnel: [w680] -> w171
    tunnel: w204 -> [w680]
    tunnel: [w679] -> w170
    tunnel: [w668] -> w168
    tunnel: [w669] -> w169
    tunnel: [w678] -> w167
    tunnel: w203 -> [w677]
    tunnel: w202 -> [w676]
    tunnel: w196 -> [w675]
    tunnel: w201 -> [w674]
    shift-right: [w667] -> _
    shift-left: _ -> [w673]
    shift-right: [w672] -> _
    shift-left: u32 0 ("New Lost") -> [w666]
    shift-right: [w671] -> w165
    shift-left: u32[] [] ("NewBuffNum") -> [w662]
    shift-right: [w670] -> w166
    shift-left: u32[] [] ("NewNumLost") -> [w663]
    tunnel: w186 -> [w661]
    tunnel: w94 -> [w659]
    i -> [w654]
    stop <- w664 stop-if-true
    n141 = call <vilib>:"IMAQdx Get Image.vi"("Buffer Number Mode (Next)"=IMAQdx_Buffer_Number_Mode."Buffer Number", "error in"=w676, "Buffer Number In"=w654, "Image In"=w675, "Session In"=w677) -> ("error out"=w687:errorcluster, "Buffer Number Out"=w667:u32, "Image Out"=w656:T1, "Session Out"=w668:T4)  [unwired: 3 in]
    "Last Whisk\nBuffer 2" <- w667
    "?" <- w656
    n142 = Greater?(x=w654, y=w659) -> (0:→"Pupil Cam":bool)
    n143 = call "TrackPupilDroppedFrames_IOS.vi"("NumLost"=w663, "BuffNum"=w662, "Curr Buffer"=w667, "Prev Lost"=w666, "Prev Buffer"=w673) -> ("New Lost"=w672:u32, "NewNumLost"=w670:u32[], "NewBuffNum"=w671:u32[])  [unwired: 4 in]
    "Dropped 2" <- w672
    n144 = call "IMAQ ImageToArray"("error in (no error)"=w687, "Image"=w656) -> ("error out"=w686:errorcluster, "Image Pixels (U8)"=w685:u8[][])  [unwired: 2 in, 3 out]
    n145 = Add(x=w667, y=w666) -> (x+y=w665:u32)
    n146 = Greater Or Equal?(x=w665, y=w661) -> ()  [unwired: 1 out]
    n147 = Write to Binary File(file (use dialog)=w674, data=w685, error in=w686, 5:FALSE ("prepend array or string size? (T)"), 9:T11."little-endian" ("byte order (0:big-endian, network order)")) -> (refnum out=w678:refnum<file>, error out=w669:errorcluster)  [unwired: 1 in, 1 out]
    n148 = local read "stop"() -> (w658:bool)
    n149 = local read "CBV Camera"() -> (w657:bool)
    n150 = call <vilib>:"Calculate Frames per Second.vi"("Update Interval (ms)"=u32 2000, "Buffer Number"=w667) -> ("Processed Frames/s"=→"Pupil Cam Fs":dbl)  [unwired: 7 in, 2 out]
    n151 = Unbundle By Name(w669) -> ("status"=w655:bool)
    n152 = Compound Arithmetic op=OR(w655, w658, w657) -> (w664:bool)
  }
  n153 = while {
    tunnel: w414 -> [w741]
    tunnel: w412 -> [w742]
    tunnel: [w724] -> w458
    tunnel: [w722] -> w459
    tunnel: [w736] -> w457
    tunnel: [w731] -> w4
    tunnel: w410 -> [w731]
    tunnel: [w730] -> w3
    tunnel: w409 -> [w730]
    tunnel: w408 -> [w729]
    tunnel: w406 -> [w728]
    tunnel: w405 -> [w727]
    tunnel: w403 -> [w721]
    tunnel: w94 -> [w716]
    tunnel: w81 -> [w711]
    tunnel: w47 -> [w699]
    tunnel: w46 -> [w700]
    tunnel: w45 -> [w694]
    tunnel: w44 -> [w691]
    i -> [w717]
    stop <- w710 stop-if-true
    n154 = Greater?(x=w717, y=w716) -> (0:→"CBV Cam":bool)
    n155 = call <vilib>:"IMAQ Extract Buffer.vi"("error in (no error)"=w742, "Buffer to extract"=w717, "IMAQ Session In"=w741) -> ("error out"=w735:errorcluster, "Buffer Number"=w712:i32, "Image Out"=w714:T1, "IMAQ Session Out"=w722:refnum<k11>)  [unwired: 5 out]
    "Last CBV\nBuffer" <- w712
    "?" <- w714
    n156 = Multiply(x=w711, y=w712) -> (x*y=w713:dbl)
    n157 = Round Toward -Infinity(1:w713) -> (0:w705:dbl)
    n158 = Tick Count (ms)() -> (millisecond timer value=w734:u32)
    n159 = call <vilib>:"Calculate Frames per Second.vi"("Update Interval (ms)"=u32 2000, "Buffer Number"=w712) -> ("Processed Frames/s"=→"CBV Cam":dbl)  [unwired: 7 in, 2 out]
    n160 = Index Array(array=w699, index (row)=w705) -> (element=w698:bool[])  [unwired: 1 in]
    n161 = Index Array(array=w700, index (row)=w705) -> (element=w696:bool[])  [unwired: 1 in]
    n162 = Index Array(array=w694, index (row)=w705) -> (element=w693:bool[])  [unwired: 1 in]
    n163 = Index Array(array=w691, index (row)=w705) -> (element=w690:bool[])  [unwired: 1 in]
    n164 = Greater Or Equal?(x=w712, y=w728) -> (x >= y?=w720:bool)
    n165 = call "IMAQ ImageToArray"("error in (no error)"=w735, "Image"=w714) -> ("error out"=w740:errorcluster, "Image Pixels (I16)"=w739:i16[][])  [unwired: 2 in, 3 out]
    n166 = Subtract(x=w734, y=w729) -> (x-y=w733:u32)
    n167 = local write "stop"("stop") -> ()
    n168 = Greater?(x=w698, y=FALSE ("Boolean")) -> (0:w697:bool[])
    n169 = Greater?(x=w696, y=FALSE ("Boolean")) -> (0:w695:bool[])
    n170 = Greater?(x=w693, y=FALSE ("Boolean")) -> (0:w692:bool[])
    n171 = Greater?(x=w690, y=FALSE ("Boolean")) -> (0:w689:bool[])
    n172 = Multiply(x=w733, y=1.667e-05) -> (x*y=w732:dbl)
    n173 = Or Array Elements(Boolean array=w697) -> (logical OR=→"LPad":bool)
    n174 = Or Array Elements(Boolean array=w695) -> (logical OR=→"Auditory":bool)
    n175 = Or Array Elements(Boolean array=w692) -> (logical OR=→"RPad":bool)
    n176 = Or Array Elements(Boolean array=w689) -> (logical OR=→"LED":bool)
    n177 = Write to Binary File(file (use dialog)=w721, data=w739, error in=w740, 5:FALSE ("prepend array or string size? (T)"), 9:T11."big-endian, network order" ("byte order (0:big-endian, network order)")) -> (refnum out=w736:refnum<file>, error out=w724:errorcluster)  [unwired: 1 in, 1 out]
    n178 = Bundle("Time (min)"=w727, w732) -> (→"Time Elapsed (Min)":cluster{"Time (min)":dbl, dbl})  [unwired: 1 in]
    n179 = Compound Arithmetic op=OR(w724, w720, "stop") -> (w710:bool)
    "CBV Camera" <- w710
    "Finished" <- w710
  }
  n180 = while {
    tunnel: w430 -> [w769]
    tunnel: [w770] -> w429
    tunnel: w428 -> [w770]
    tunnel: [w769] -> w427
    tunnel: [w762] -> w292
    tunnel: [w763] -> w349
    tunnel: [w768] -> w426
    tunnel: w425 -> [w767]
    tunnel: w423 -> [w766]
    tunnel: w421 -> [w765]
    tunnel: w419 -> [w764]
    shift-right: [w753] -> _
    shift-left: _ -> [w751]
    shift-right: [w748] -> _
    shift-left: u32 0 ("New Lost") -> [w752]
    shift-right: [w749] -> w284
    shift-left: u32[] [] ("NewBuffNum") -> [w750]
    shift-right: [w755] -> w373
    shift-left: u32[] [] ("NewNumLost") -> [w754]
    tunnel: w187 -> [w760]
    tunnel: w94 -> [w756]
    i -> [w743]
    stop <- w759 stop-if-true
    n181 = call <vilib>:"IMAQdx Get Image.vi"("Buffer Number Mode (Next)"=IMAQdx_Buffer_Number_Mode."Buffer Number", "error in"=w766, "Buffer Number In"=w743, "Image In"=w765, "Session In"=w767) -> ("error out"=w776:errorcluster, "Buffer Number Out"=w753:u32, "Image Out"=w745:T1, "Session Out"=w762:T4)  [unwired: 3 in]
    "Last Whisk\nBuffer" <- w753
    "?" <- w745
    n182 = Greater?(x=w743, y=w756) -> (0:→"Whisk Cam":bool)
    n183 = call "IMAQ ImageToArray"("error in (no error)"=w776, "Image"=w745) -> ("error out"=w775:errorcluster, "Image Pixels (U8)"=w774:u8[][])  [unwired: 2 in, 3 out]
    n184 = call "TrackWhiskDroppedFrames_IOS.vi"("NumLost"=w754, "BuffNum"=w750, "Curr Buffer"=w753, "Prev Lost"=w752, "Prev Buffer"=w751) -> ("New Lost"=w748:u32, "NewNumLost"=w755:u32[], "NewBuffNum"=w749:u32[])  [unwired: 4 in]
    "Dropped" <- w748
    n185 = Add(x=w753, y=w752) -> (x+y=w761:u32)
    n186 = Greater Or Equal?(x=w761, y=w760) -> ()  [unwired: 1 out]
    n187 = Write to Binary File(file (use dialog)=w764, data=w774, error in=w775, 5:FALSE ("prepend array or string size? (T)"), 9:T11."little-endian" ("byte order (0:big-endian, network order)")) -> (refnum out=w768:refnum<file>, error out=w763:errorcluster)  [unwired: 1 in, 1 out]
    n188 = local read "stop"() -> (w747:bool)
    n189 = local read "CBV Camera"() -> (w746:bool)
    n190 = call <vilib>:"Calculate Frames per Second.vi"("Update Interval (ms)"=u32 2000, "Buffer Number"=w753) -> ("Processed Frames/s"=→"Whisk Cam Fs":dbl)  [unwired: 7 in, 2 out]
    n191 = Unbundle By Name(w763) -> ("status"=w744:bool)
    n192 = Compound Arithmetic op=OR(w744, w747, w746) -> (w759:bool)
  }
  n193 = while {
    tunnel: w446 -> [w794]
    tunnel: w440 -> [w792]
    tunnel: w438 -> [w791]
    tunnel: w436 -> [w790]
    tunnel: w433 -> [w788]
    tunnel: [w789] -> w200
    tunnel: [w780] -> w431
    tunnel: [w788] -> w432
    tunnel: w94 -> [w783]
    i -> [w784]
    stop <- w781 stop-if-true
    n194 = Tick Count (ms)() -> (millisecond timer value=w796:u32)
    n195 = Subtract(x=w796, y=w794) -> (x-y=w797:u32)
    n196 = Divide(x=w797, y=u32 1000) -> (x/y=w793:dbl)
    n197 = Greater?(x=w784, y=w783) -> (0:→"Web Cam":bool)
    n198 = call "GrabWebCam_IOS.vi"("Session In"=w791, "Image In"=w792, "Trial Time"=w793, "AVI Refnum"=w788, "error in"=w790) -> ("Session Out"=w789:T4, "WebCam Img Out"=→"?":T1, "Buffer Number Out"=w787:u32, "error out"=w780:errorcluster)  [unwired: 7 in]
    n199 = local read "CBV Camera"() -> (w782:bool)
    n200 = local read "stop"() -> (w779:bool)
    n201 = call <vilib>:"Calculate Frames per Second.vi"("Update Interval (ms)"=u32 5000, "Buffer Number"=w787) -> ("Processed Frames/s"=→"Web Cam Fs":dbl)  [unwired: 7 in, 2 out]
    n202 = Compound Arithmetic op=OR(w780, w779, w782) -> (w781:bool)
  }
  n203 = while {
    tunnel: w391 -> [w821]
    tunnel: w390 -> [w820]
    tunnel: w122 -> [w819]
    tunnel: [w818] -> w160
    tunnel: [w807] -> w159
    tunnel: [w817] -> w387
    shift-right: [w811] -> _
    shift-left: w94 -> [w802]
    tunnel: [w807] -> w250
    tunnel: w123 -> [w805]
    i -> [w803]
    stop <- w808 stop-if-true
    n204 = To Long Integer(number=w805) -> (32bit integer=w806:i32)
    n205 = call-poly <vilib>:"DAQmx Read.vi"("task/channels in"=w820, "error in"=w821) -> ("task out"=w817:refnum<k21>, "data"=w799:waveform(dbl)[], "error out"=w810:errorcluster)  [unwired: 11 in]
    n206 = Greater?(x=w802, y=w803) -> (0:→"Dev1 Analog":bool)
    n207 = TDMS Write(0:w819, 5:"Analog Data" ("group name in (Untitled)"), 9:w799, 11:w810) -> (4:w818:refnum<k34>, 15:w807:errorcluster)  [unwired: 2 in, 2 out]
    n208 = Index Array(array=w799, index=0) -> (element=w814:waveform(dbl))
    n209 = Unbundle By Name(w814) -> ("Y"=w813:dbl[])
    n210 = local read "CBV Camera"() -> (w801:bool)
    n211 = local read "stop"() -> (w800:bool)
    n212 = Array Size(array=w813) -> (size(s)=w812:i32)
    n213 = Add(x=w812, y=w802) -> (x+y=w811:i32)
    "Dev1 Samples" <- w811
    n214 = Greater Or Equal?(x=w811, y=w806) -> (x >= y?=w809:bool)
    n215 = Compound Arithmetic op=OR(w807, w809, w800, w801) -> (w808:bool)
  }
  n216 = while {
    tunnel: w120 -> [w844]
    tunnel: w121 -> [w843]
    tunnel: [w842] -> w106
    tunnel: [w831] -> w107
    tunnel: [w841] -> w117
    shift-right: [w835] -> _
    shift-left: w94 -> [w826]
    tunnel: [w831] -> w116
    tunnel: w123 -> [w829]
    tunnel: w97 -> [w823]
    i -> [w827]
    stop <- w832 stop-if-true
    n217 = To Long Integer(number=w829) -> (32bit integer=w830:i32)
    n218 = call-poly <vilib>:"DAQmx Read.vi"("task/channels in"=w843, "error in"=w844) -> ("task out"=w841:refnum<k21>, "data"=w822:waveform(dbl)[], "error out"=w834:errorcluster)  [unwired: 11 in]
    n219 = Greater?(x=w826, y=w827) -> (0:→"Dev2 Analog":bool)
    n220 = TDMS Write(0:w823, 5:"Analog Data" ("group name in (Untitled)"), 9:w822, 11:w834) -> (4:w842:refnum<k34>, 15:w831:errorcluster)  [unwired: 2 in, 2 out]
    n221 = Index Array(array=w822, index=0) -> (element=w838:waveform(dbl))
    n222 = Unbundle By Name(w838) -> ("Y"=w837:dbl[])
    n223 = local read "CBV Camera"() -> (w825:bool)
    n224 = local read "stop"() -> (w824:bool)
    n225 = Array Size(array=w837) -> (size(s)=w836:i32)
    n226 = Add(x=w836, y=w826) -> (x+y=w835:i32)
    "Dev2 Samples" <- w835
    n227 = Greater Or Equal?(x=w835, y=w830) -> (x >= y?=w833:bool)
    n228 = Compound Arithmetic op=OR(w831, w833, w824, w825) -> (w832:bool)
  }
  n229 = while {
    tunnel: w22 -> [w845]
    tunnel: [w846] -> w7
    tunnel: w21 -> [w846]
    tunnel: [w845] -> w8
    stop <- w847 stop-if-true
    n230 = local read "Finished"() -> (w847:bool)
  }
  n231 = call <vilib>:"DAQmx Stop Task.vi"("task/channels in"=w117, "error in"=w116) -> ("task out"=w119:refnum<k21>, "error out"=w118:errorcluster)  [unwired: 12 in]
  n232 = call <vilib>:"DAQmx Stop Task.vi"("task/channels in"=w387, "error in"=w250) -> ("task out"=w351:refnum<k21>, "error out"=w350:errorcluster)  [unwired: 12 in]
  n233 = flat-sequence {
    tunnel: w8 -> [w855]
    tunnel: w7 -> [w854]
    tunnel: [w853] -> w6
    tunnel: [w852] -> w5
    tunnel: w4 -> [w851]
    tunnel: w3 -> [w850]
    tunnel: [w849] -> w2
    tunnel: [w848] -> w1
    tunnel: w6 -> [w859]
    tunnel: w5 -> [w858]
    tunnel: w2 -> [w857]
    tunnel: w1 -> [w856]
    frame #0 {
      n234 = call <vilib>:"DAQmx Stop Task.vi"("task/channels in"=w851, "error in"=w850) -> ("task out"=w849:refnum<k21>, "error out"=w848:errorcluster)  [unwired: 12 in]
      n235 = call <vilib>:"DAQmx Stop Task.vi"("task/channels in"=w855, "error in"=w854) -> ("task out"=w853:refnum<k21>, "error out"=w852:errorcluster)  [unwired: 12 in]
    }
    frame #1 {
      n236 = call <vilib>:"DAQmx Clear Task.vi"("task in"=w857, "error in"=w856) -> ()  [unwired: 13 in, 1 out]
      n237 = call <vilib>:"DAQmx Clear Task.vi"("task in"=w859, "error in"=w858) -> ()  [unwired: 13 in, 1 out]
    }
  }
  n238 = call <vilib>:"IMAQ Extract Buffer.vi"("error in (no error)"=w458, "Buffer to extract"=-1, "IMAQ Session In"=w459) -> ("error out"=w480:errorcluster, "IMAQ Session Out"=w479:refnum<k11>)  [unwired: 7 out]
  n239 = Close File(refnum=w457, error in=w159) -> (path=w367:path)  [unwired: 1 out]
  n240 = Delete From Array(array=w284, length=1, index=0) -> (array with subset deleted=w261:u32[])  [unwired: 1 out]
  n241 = Delete From Array(array=w373, length=1, index=0) -> (array with subset deleted=w262:u32[])  [unwired: 1 out]
  n242 = call <vilib>:"DAQmx Stop Task.vi"("task/channels in"=w170, "error in"=w171) -> ("task out"=w153:refnum<k21>, "error out"=w154:errorcluster)  [unwired: 12 in]
  n243 = call <vilib>:"DAQmx Stop Task.vi"("task/channels in"=w427, "error in"=w429) -> ("task out"=w151:refnum<k21>, "error out"=w152:errorcluster)  [unwired: 12 in]
  n244 = Delete From Array(array=w166, length=1, index=0) -> (array with subset deleted=w173:u32[])  [unwired: 1 out]
  n245 = Delete From Array(array=w165, length=1, index=0) -> (array with subset deleted=w172:u32[])  [unwired: 1 out]
  n246 = call <vilib>:"IMAQdx Close Camera.vi"("error in"=w349, "Session In"=w292) -> ()  [unwired: 9 in, 1 out]
  n247 = Close File(refnum=w426, error in=w349) -> (path=w365:path, error out=w364:errorcluster)
  n248 = call "IMAQ AVI2 Close"("error in (no error)"=w431, "AVI Refnum"=w432) -> ("error out"=w366:errorcluster)  [unwired: 9 in]
  n249 = call <vilib>:"IMAQdx Close Camera.vi"("error in"=w431, "Session In"=w200) -> ()  [unwired: 9 in, 1 out]
  n250 = call <vilib>:"DAQmx Clear Task.vi"("task in"=w119, "error in"=w118) -> ()  [unwired: 13 in, 1 out]
  n251 = call <vilib>:"IMAQdx Close Camera.vi"("error in"=w169, "Session In"=w168) -> ()  [unwired: 9 in, 1 out]
  n252 = Close File(refnum=w167, error in=w169) -> (path=w162:path, error out=w161:errorcluster)
  n253 = Build Array(w261, w262) -> (w264:u32[][])
  n254 = call <vilib>:"DAQmx Clear Task.vi"("task in"=w351, "error in"=w350) -> ()  [unwired: 13 in, 1 out]
  n255 = call <vilib>:"IMAQ Close.vi"("error in (no error)"=w480, "IMAQ Session In"=w479) -> ("error out"=w481:errorcluster)  [unwired: 9 out]
  n256 = Build Array(w172, w173) -> (w175:u32[][])
  n257 = call <vilib>:"DAQmx Clear Task.vi"("task in"=w151, "error in"=w152) -> ()  [unwired: 13 in, 1 out]
  n258 = call <vilib>:"DAQmx Clear Task.vi"("task in"=w153, "error in"=w154) -> ()  [unwired: 13 in, 1 out]
  n259 = Array To Spreadsheet String(delimiter (Tab)=",", array=w262, 3:"%d" ("format string")) -> (spreadsheet string=w285:string)
  n260 = Transpose 2D Array(2D array=w264) -> (transposed array=w263:u32[][])
  n261 = Array To Spreadsheet String(delimiter (Tab)=",", array=w261, 3:"%d" ("format string")) -> (spreadsheet string=w286:string)
  n262 = Move(source path=w162, error in=w161, 10:"Target Path") -> (error out=w163:errorcluster)  [unwired: 2 in, 2 out]
  n263 = Move(source path=w365, error in=w364, 10:"Target Path") -> (error out=w362:errorcluster)  [unwired: 2 in, 2 out]
  n264 = Array To Spreadsheet String(delimiter (Tab)=",", array=w173, 3:"%d" ("format string")) -> (spreadsheet string=w176:string)
  n265 = Transpose 2D Array(2D array=w175) -> (transposed array=w174:u32[][])
  n266 = Array To Spreadsheet String(delimiter (Tab)=",", array=w172, 3:"%d" ("format string")) -> (spreadsheet string=w177:string)
  n267 = Move(source path=w79, error in=w366, 10:"Target Path") -> (error out=w361:errorcluster)  [unwired: 2 in, 2 out]
  n268 = TDMS Close(8:w107, 11:w106) -> (0:w115:errorcluster, 3:w95:path)
  n269 = for {
    N: w32 -> [_]
    tunnel: w475 -> [w863] mode=indexing
    shift-right: [w861] -> w369
    shift-left: w481 -> [w862]
    n270 = call "IMAQ Dispose"("All Images? (No)"=FALSE, "Image"=w863, "error in (no error)"=w862) -> ("error out"=w861:errorcluster)  [unwired: 3 out]
  }
  n271 = call <vilib>:"Trim Whitespace.vi"("string"=w286) -> ("trimmed string"=w147:string)  [unwired: 1 in]
  n272 = call <vilib>:"Trim Whitespace.vi"("string"=w285) -> ("trimmed string"=w146:string)  [unwired: 1 in]
  n273 = Number To Decimal String(number=w263) -> ()  [unwired: 1 in, 1 out]
  n274 = call <vilib>:"Trim Whitespace.vi"("string"=w177) -> ("trimmed string"=w148:string)  [unwired: 1 in]
  n275 = call <vilib>:"Trim Whitespace.vi"("string"=w176) -> ("trimmed string"=w149:string)  [unwired: 1 in]
  n276 = Number To Decimal String(number=w174) -> ()  [unwired: 1 in, 1 out]
  n277 = call <vilib>:"Simple Error Handler.vi"("error in (no error)"=w163) -> ()  [unwired: 1 in, 8 out]
  n278 = call <vilib>:"Simple Error Handler.vi"("error in (no error)"=w362) -> ()  [unwired: 1 in, 8 out]
  n279 = Path To String(path=w95) -> (string=w113:string)
  n280 = call <vilib>:"Simple Error Handler.vi"("error in (no error)"=w361) -> ()  [unwired: 1 in, 8 out]
  n281 = TDMS Defragment(4:w115, 7:w95) -> (0:w109:errorcluster)
  n282 = Build Array(w148, w149, w147, w146) -> (w145:string[])
  n283 = Concatenate Strings(w113, "_index" ("string")) -> (w111:string)
  n284 = Move(source path=w367, error in=w369, 10:"Target Path") -> (error out=w368:errorcluster)  [unwired: 2 in, 2 out]
  n285 = String To Path(string=w111) -> (path=w110:path)
  n286 = call <vilib>:"Simple Error Handler.vi"("error in (no error)"=w368) -> ()  [unwired: 1 in, 8 out]
  n287 = Move(source path=w95, error in=w109, 10:"Target Path") -> (error out=w114:errorcluster)  [unwired: 2 in, 2 out]
  n288 = Move(source path=w110, error in=w109, 10:"Target Path") -> (error out=w108:errorcluster)  [unwired: 2 in, 2 out]
  n289 = TDMS Set Properties(5:w145, 7:string[] ["PupilCam_DroppedFrameIndex", "PupilCam_NumberDropped", "WhiskCam_DroppedFrameIndex", "WhiskCam_NumberDropped"] ("channel name(s) in (Untitled)"), 8:w159, 11:w160) -> (0:w293:errorcluster, 3:w291:refnum<k34>)  [unwired: 2 in, 2 out]
  n290 = call <vilib>:"Simple Error Handler.vi"("error in (no error)"=w114) -> ()  [unwired: 1 in, 8 out]
  n291 = call <vilib>:"Simple Error Handler.vi"("error in (no error)"=w108) -> ()  [unwired: 1 in, 8 out]
  n292 = TDMS Close(8:w293, 11:w291) -> (0:w370:errorcluster, 3:w358:path)
  n293 = Path To String(path=w358) -> (string=w360:string)
  n294 = TDMS Defragment(4:w370, 7:w358) -> (0:w355:errorcluster)
  n295 = Concatenate Strings(w360, "_index" ("string")) -> (w357:string)
  n296 = String To Path(string=w357) -> (path=w356:path)
  n297 = Move(source path=w358, error in=w355, 10:"Target Path") -> (error out=w363:errorcluster)  [unwired: 2 in, 2 out]
  n298 = Move(source path=w356, error in=w355, 10:"Target Path") -> (error out=w164:errorcluster)  [unwired: 2 in, 2 out]
  n299 = call <vilib>:"Simple Error Handler.vi"("error in (no error)"=w363) -> ()  [unwired: 1 in, 8 out]
  n300 = call <vilib>:"Simple Error Handler.vi"("error in (no error)"=w164) -> ()  [unwired: 1 in, 8 out]
